vi "ODrive velocity control and error managment.vi"(8 "error in (no error)":errorcluster, 11 "Refnum in":refnum<k20>) -> (0 "Error out":errorcluster, 3 "Refnum out":refnum<k20>)   [LabVIEW 2016]
uses:
  Typedef/Remote Control Cluster.ctl
  Shared resoruces/Front Panel Control Variables.vi
  <vilib>/Utility/error.llb/Error Cluster From Error Code.vi
  <vilib>/rvi/errors/niLvFpgaAdjustHostInterfaceError.vi
  <vilib>/RVI Host/nirviSupport.llb/nirviErrorClusterFromErrorCode.vi
  <vilib>/rvi/interface/nirviMethod/nirviMethod.xnode
  <vilib>/rvi/interface/nirviReadWriteControl/nirviReadWriteControl.xnode
  <vilib>/FPGAPlugInAG/Dynamic/niLvFpga_WriteFifo_Dynamic.vi
  <vilib>/rvi/errors/niLvFpgaMergeErrorWithErrorCode.vi
  Shared resoruces/Shared resources RT.lvlib
  NiFpgaLv.dll
  <vilib>/rvi/interface/Simulation/niFpgaSimulationCallBeginRW.vi
  <vilib>/rvi/interface/nirviMethod/StockFPGA_InlinedMethodWaitForSingleIRQ.vi
  <vilib>/FPGAPlugInAG/Dynamic/niLvFpga_WaitOnIrq_Dynamic.vi
  <vilib>/FPGAPlugInAG/Dynamic/niLvFpga_AcknowledgeIrq_Dynamic.vi
panel:
  in  "maxDiff":i16=5
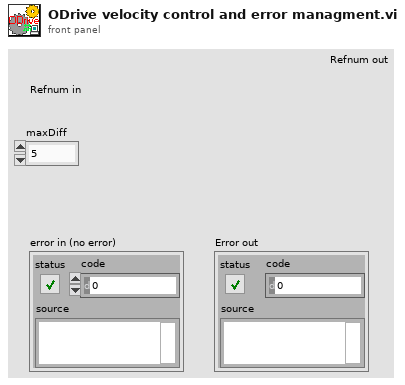
[diagram p1: front panel]
types:
  T1 = typedef "Remote Control Cluster.ctl" = cluster{"Pot1":u16, "Pot2":u16, "Pot3":u16, "Pot4":u16, "Switch1":cluster{"L":bool, "H":bool}, "Switch2":cluster{"L":bool, "H":bool}, "Switch3":cluster{"L":bool, "H":bool}}
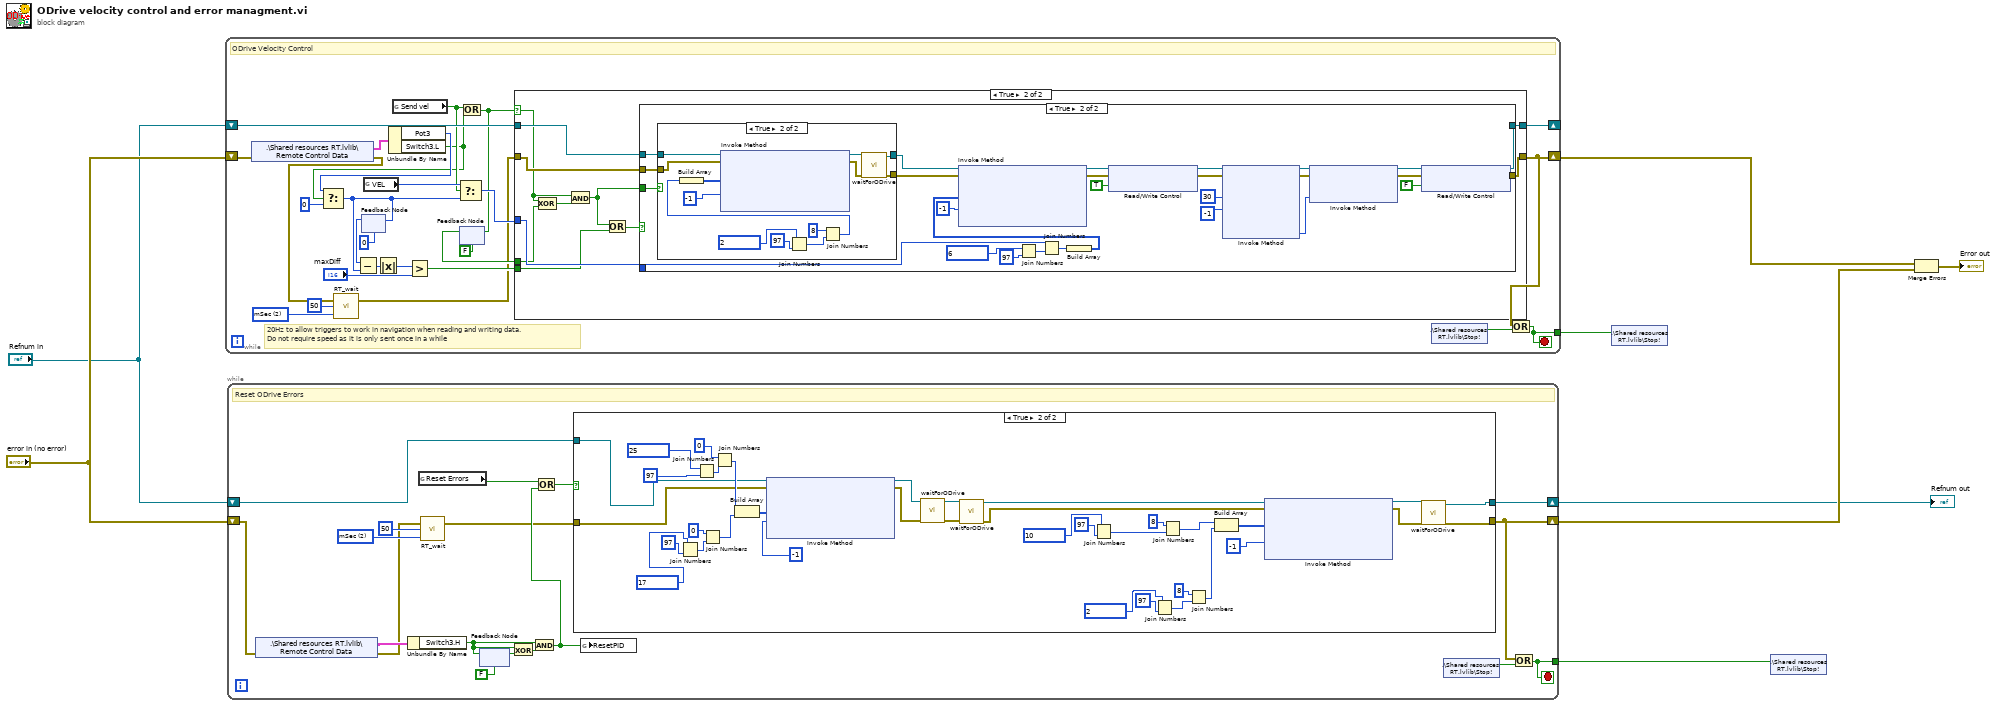
[diagram p0: block diagram]
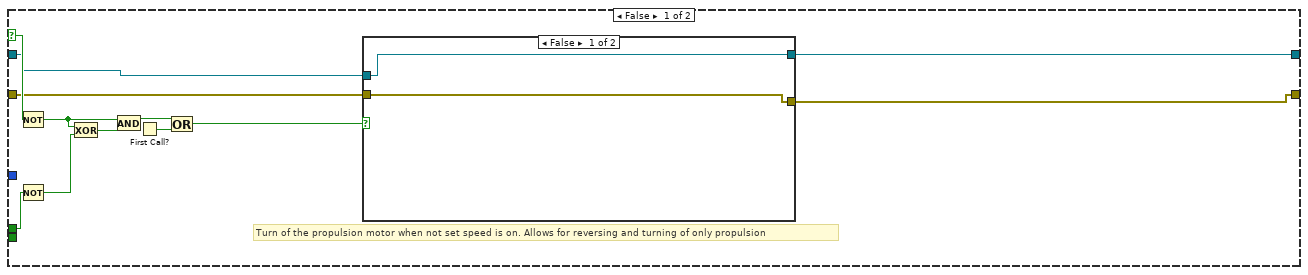
[diagram p2: hidden frame]
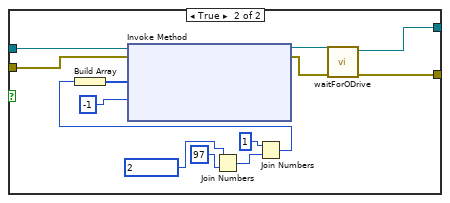
[diagram p3: hidden frame]
diagram:
  n1 = while {
    shift-right: [w35] -> _
    shift-left: "Refnum in" -> [w34]
    shift-right: [w30] -> w3
    shift-left: "error in (no error)" -> [w33]
    tunnel: [w29] -> w6
    stop <- w29 stop-if-true
    w11 = u16 2 items=["Ticks", "uSec", "mSec"] ("Counter Units")
    # "20Hz to allow triggers to work in navigation when reading and writing data. \nDo not require speed as it is only sent once in a while"
    # "ODrive Velocity Control"
    n2 = shared-variable ".\\Shared resources RT.lvlib\\Remote Control Data"(error in=w33) -> (w32:T1, error out=w10:errorcluster)
    n3 = call "RT_wait.vi"("Counter Units"=w11, "Count(mSec)"=u32 50, "error in (no error)"=w10) -> ("error out"=w9:errorcluster)  [unwired: 1 in, 1 out]
    n4 = feedback #1(u16 0) -> (w24:u16)
    n5 = global read "Front Panel Control Variables.vi" "VEL"() -> (w27:u16)
    n6 = Unbundle By Name(w32) -> ("Pot3"=w18:u16, "Switch3.L"=w17:bool)
    n7 = Select(t=w18, s=w17, f=u16 0) -> (s? t:f=w19:u16)
    n8 = Subtract(x=w24, y=w19) -> (x-y=w23:i16)
    n9 = feedback-in #1(w19) -> ()
    n10 = Absolute Value(x=w23) -> (abs(x)=w22:i16)
    n11 = global read "Front Panel Control Variables.vi" "Send vel"() -> (w26:bool)
    n12 = Greater?(x=w22, y="maxDiff") -> (0:w14:bool)
    n13 = Select(t=w27, s=w26, f=w19) -> (s? t:f=w28:u16)
    n14 = Or(x=w26, y=w17) -> (x .or. y?=w13:bool)
    n15 = feedback-in #2(w13) -> ()
    n16 = feedback #2(FALSE) -> (w15:bool)
    n17 = case shown="True" w13 {
      selector: w13 -> [w45 w67]
      tunnel: w28 -> [_ w73]
      tunnel: [w42 w72] -> w30
      tunnel: [w41 w71] -> w35
      tunnel: w9 -> [w43 w70]
      tunnel: w34 -> [w44 w69]
      tunnel: w15 -> [w36 w66]
      tunnel: w14 -> [_ w65]
      frame False {
        # "Turn of the propulsion motor when not set speed is on. Allows for reversing and turning of only propulsion"
        n18 = Not(x=w45) -> (.not. x?=w46:bool)
        n19 = Not(x=w36) -> (.not. x?=w39:bool)
        n20 = Exclusive Or(1:w39, 2:w46) -> (0:w47:bool)
        n21 = And(x=w46, y=w47) -> (x .and. y?=w40:bool)
        n22 = First Call?() -> (First Call?: T/F=w37:bool)
        n23 = Or(x=w40, y=w37) -> (x .or. y?=w38:bool)
        n24 = case shown="False" w38 {
          tunnel: w44 -> [w48 w53]
          tunnel: w43 -> [w49 w52]
          tunnel: [w49 w51] -> w42
          tunnel: [w48 w50] -> w41
          frame False {
          }
          frame True {
            n25 = Join Numbers(hi=u8 2 ("lo"), lo=u8 97) -> ((hi.lo)=w60:u16)
            n26 = Join Numbers(hi=u16 1, lo=w60) -> ((hi.lo)=w57:u32)
            n27 = Build Array(w57) -> (w62:u32[])
            n28 = xnode "Invoke Method"("FPGA VI Reference In"=w53, "error in"=w52, "Data"=w62, "Timeout (ms)"=-1) -> ("FPGA VI Reference Out"=w55:refnum<k20>, "error out"=w54:errorcluster)  [unwired: 1 out]
            n29 = call "waitForODrive.vi"("error in (no error)"=w54, "Refnum in"=w55) -> ("error out"=w51:errorcluster, "Refnum out"=w50:refnum<k20>)  [unwired: 8 in]
          }
        }
      }
      frame True {
        n30 = Exclusive Or(1:w66, 2:w67) -> (0:w68:bool)
        n31 = And(x=w67, y=w68) -> (x .and. y?=w63:bool)
        n32 = Or(x=w63, y=w65) -> (x .or. y?=w64:bool)
        n33 = case shown="True" w64 {
          tunnel: w73 -> [_ w83]
          tunnel: [w75 w82] -> w72
          tunnel: [w74 w81] -> w71
          tunnel: w70 -> [w75 w79]
          tunnel: w69 -> [w74 w78]
          tunnel: w63 -> [_ w76]
          frame False {
          }
          frame True {
            n34 = case shown="True" w76 {
              tunnel: w78 -> [w103 w108]
              tunnel: w79 -> [w104 w107]
              tunnel: [w104 w106] -> w80
              tunnel: [w103 w105] -> w77
              frame False {
              }
              frame True {
                n35 = Join Numbers(hi=u8 2 ("lo"), lo=u8 97) -> ((hi.lo)=w115:u16)
                n36 = Join Numbers(hi=u16 8, lo=w115) -> ((hi.lo)=w112:u32)
                n37 = Build Array(w112) -> (w117:u32[])
                n38 = xnode "Invoke Method"("FPGA VI Reference In"=w108, "error in"=w107, "Data"=w117, "Timeout (ms)"=-1) -> ("FPGA VI Reference Out"=w110:refnum<k20>, "error out"=w109:errorcluster)  [unwired: 1 out]
                n39 = call "waitForODrive.vi"("error in (no error)"=w109, "Refnum in"=w110) -> ("error out"=w106:errorcluster, "Refnum out"=w105:refnum<k20>)  [unwired: 8 in]
              }
            }
            n40 = Join Numbers(hi=u8 6 ("lo"), lo=u8 97) -> ((hi.lo)=w87:u16)
            n41 = Join Numbers(hi=w83, lo=w87) -> ((hi.lo)=w86:u32)
            n42 = Build Array(w86) -> (w84:u32[])
            n43 = xnode "Invoke Method"("FPGA VI Reference In"=w77, "error in"=w80, "Data"=w84, "Timeout (ms)"=-1) -> ("FPGA VI Reference Out"=w91:refnum<k20>, "error out"=w92:errorcluster)  [unwired: 1 out]
            n44 = xnode "Read/Write Control"("FPGA VI Reference In"=w91, "error in"=w92, "ODrive RT Control"=TRUE) -> ("FPGA VI Reference Out"=w90:refnum<k20>, "error out"=w89:errorcluster)
            n45 = xnode "Invoke Method"("FPGA VI Reference In"=w90, "error in"=w89, "IRQ Number(s)"=30, "Timeout (ms)"=-1) -> ("FPGA VI Reference Out"=w101:refnum<k20>, "error out"=w98:errorcluster, "IRQ(s) Asserted"=w99:i32)  [unwired: 1 out]
            n46 = xnode "Invoke Method"("FPGA VI Reference In"=w101, "error in"=w98, "IRQ Number(s)"=w99) -> ("FPGA VI Reference Out"=w96:refnum<k20>, "error out"=w95:errorcluster)
            n47 = xnode "Read/Write Control"("FPGA VI Reference In"=w96, "error in"=w95, "ODrive RT Control"=FALSE) -> ("FPGA VI Reference Out"=w81:refnum<k20>, "error out"=w82:errorcluster)
          }
        }
      }
    }
    n48 = shared-variable ".\\Shared resources RT.lvlib\\Stop!"() -> (w31:bool)  [unwired: 1 in, 1 out]
    n49 = Or(x=w30, y=w31) -> (x .or. y?=w29:bool)
  }
  n50 = while {
    shift-right: [w134] -> w1
    shift-left: "Refnum in" -> [w135]
    shift-right: [w129] -> w4
    shift-left: "error in (no error)" -> [w131]
    tunnel: [w128] -> w5
    stop <- w128 stop-if-true
    w121 = u16 2 items=["Ticks", "uSec", "mSec"] ("Counter Units")
    # "Reset ODrive Errors"
    n51 = shared-variable ".\\Shared resources RT.lvlib\\Remote Control Data"(error in=w131) -> (w132:T1, error out=w119:errorcluster)
    n52 = Unbundle By Name(w132) -> ("Switch3.H"=w123:bool)
    n53 = global read "Front Panel Control Variables.vi" "Reset Errors"() -> (w127:bool)
    n54 = call "RT_wait.vi"("Counter Units"=w121, "Count(mSec)"=u32 50, "error in (no error)"=w119) -> ("error out"=w118:errorcluster)  [unwired: 1 in, 1 out]
    n55 = feedback #3(FALSE) -> (w124:bool)
    n56 = feedback-in #3(w123) -> ()
    n57 = Exclusive Or(1:w124, 2:w123) -> (0:w126:bool)
    n58 = And(x=w123, y=w126) -> (x .and. y?=w122:bool)
    n59 = Or(x=w127, y=w122) -> (x .or. y?=w133:bool)
    n60 = case shown="True" w133 {
      tunnel: w135 -> [w137 w157]
      tunnel: w118 -> [w136 w156]
      tunnel: [w137 w139] -> w134
      tunnel: [w136 w138] -> w129
      frame False {
      }
      frame True {
        n61 = Join Numbers(hi=u8 17 ("lo"), lo=u8 97) -> ((hi.lo)=w162:u16)
        n62 = Join Numbers(hi=u8 25 ("lo"), lo=u8 97) -> ((hi.lo)=w173:u16)
        n63 = Join Numbers(hi=u16 0, lo=w162) -> ((hi.lo)=w160:u32)
        n64 = Join Numbers(hi=u16 0, lo=w173) -> ((hi.lo)=w171:u32)
        n65 = Build Array(w171, w160) -> (w170:u32[])
        n66 = xnode "Invoke Method"("FPGA VI Reference In"=w157, "error in"=w156, "Data"=w170, "Timeout (ms)"=-1) -> ("FPGA VI Reference Out"=w167:refnum<k20>, "error out"=w168:errorcluster)  [unwired: 1 out]
        n67 = call "waitForODrive.vi"("error in (no error)"=w168, "Refnum in"=w167) -> ("error out"=w159:errorcluster, "Refnum out"=w158:refnum<k20>)  [unwired: 8 in]
        n68 = call "waitForODrive.vi"("error in (no error)"=w159, "Refnum in"=w158) -> ("error out"=w142:errorcluster, "Refnum out"=w143:refnum<k20>)  [unwired: 8 in]
        n69 = Join Numbers(hi=u8 10 ("lo"), lo=u8 97) -> ((hi.lo)=w152:u16)
        n70 = Join Numbers(hi=u8 2 ("lo"), lo=u8 97) -> ((hi.lo)=w148:u16)
        n71 = Join Numbers(hi=u16 8, lo=w152) -> ((hi.lo)=w154:u32)
        n72 = Join Numbers(hi=u16 8, lo=w148) -> ((hi.lo)=w145:u32)
        n73 = Build Array(w154, w145) -> (w155:u32[])
        n74 = xnode "Invoke Method"("FPGA VI Reference In"=w143, "error in"=w142, "Data"=w155, "Timeout (ms)"=-1) -> ("FPGA VI Reference Out"=w141:refnum<k20>, "error out"=w140:errorcluster)  [unwired: 1 out]
        n75 = call "waitForODrive.vi"("error in (no error)"=w140, "Refnum in"=w141) -> ("error out"=w138:errorcluster, "Refnum out"=w139:refnum<k20>)  [unwired: 8 in]
      }
    }
    n76 = global write "Front Panel Control Variables.vi" "ResetPID"(w122) -> ()
    n77 = shared-variable ".\\Shared resources RT.lvlib\\Stop!"() -> (w130:bool)  [unwired: 1 in, 1 out]
    n78 = Or(x=w129, y=w130) -> (x .or. y?=w128:bool)
  }
  "Refnum out" <- w1
  n79 = shared-variable ".\\Shared resources RT.lvlib\\Stop!"(w6) -> ()  [unwired: 1 in, 1 out]
  n80 = shared-variable ".\\Shared resources RT.lvlib\\Stop!"(w5) -> ()  [unwired: 1 in, 1 out]
  n81 = Merge Errors(w3, w4) -> (→"Error out":errorcluster)
